vi "AN97005H-ONOFF.vi"(8 "error in":errorcluster caption="错误输入（无错误）", 10 "模式":enum16{"启动", "停止"}(ring), 11 "MyIndex":u8) -> (0 "error out":errorcluster caption="错误输出", 3 "OK?":bool)   [LabVIEW 2015, in "AN97005N.lvlib"]
uses:
  AN97005N.lvlib
  <vilib>/Instr/_visa.llb/VISA Configure Serial Port (Instr).vi
panel:
  out "AC电源":refnum<visa-resource-name>
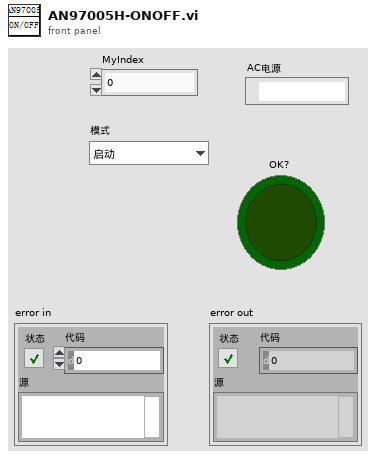
[diagram p1: front panel]
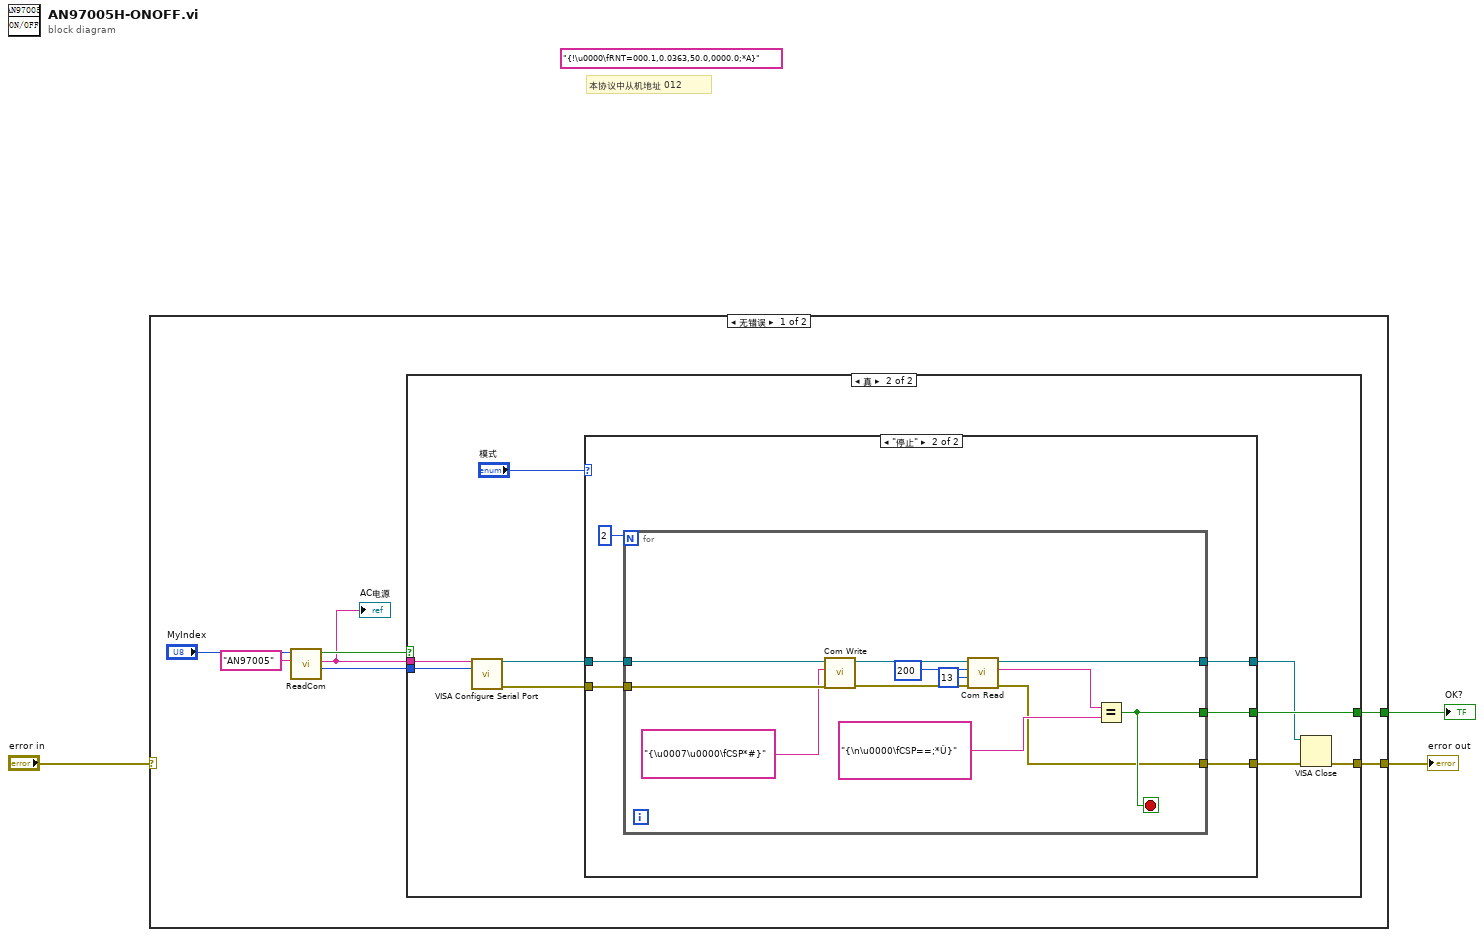
[diagram p0: block diagram]
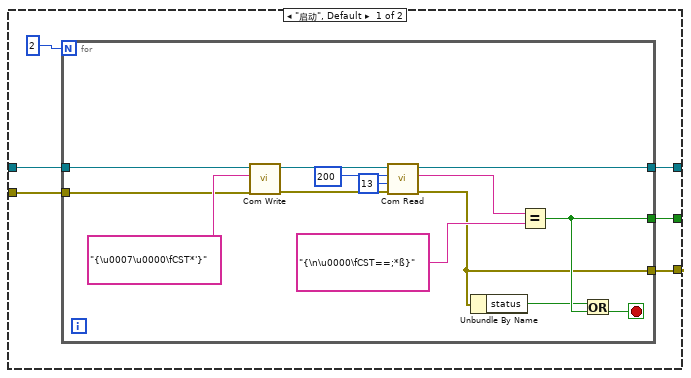
[diagram p3: hidden frame]
diagram:
  (unwired) "{!\u0000\fRNT=000.1,0.0363,50.0,0000.0;*A}"
  # "本协议中从机地址 012"
  n1 = case shown="无错误" "error in" {
    selector: "error in" -> [_ w58]
    tunnel: [w10 _] -> w3
    tunnel: [w4 w58] -> w2
    frame No Error {
      n2 = call "ReadCom.vi"("仪器名称"="AN97005", "MyIndex"="MyIndex") -> ("Baudrate"=w6:i32, "COM"=w5:string, "OK?"=w7:bool)  [unwired: 7 in]
      "AC电源" <- w5
      n3 = case shown="真" w7 {
        tunnel: [_ w18] -> w10
        tunnel: [_ w14] -> w4
        tunnel: w5 -> [_ w16]
        tunnel: w6 -> [_ w11]
        frame False {
        }
        frame True {
          n4 = call-poly "VISA Configure Serial Port"("VISA resource name"=w16, "baud rate (9600)"=w11) -> ("VISA resource name out"=w15:refnum<visa-resource-name>, "error out"=w12:errorcluster)  [unwired: 12 in]
          n5 = case shown="\"停止\"" "模式" {
            tunnel: w15 -> [w25 w45]
            tunnel: [w23 w43] -> w18
            tunnel: [w22 w42] -> w17
            tunnel: [w21 w41] -> w13
            tunnel: w12 -> [w20 w40]
            frame "启动", Default {
              n6 = for {
                N: 2 -> [_]
                tunnel: [w30] -> w23
                tunnel: [w29] -> w22
                tunnel: w25 -> [w39]
                tunnel: [w33] -> w21
                tunnel: w20 -> [w26]
                stop <- w28 stop-if-true
                n7 = call "Com Write.vi"("错误输入（无错误）"=w26, "Wbuff"="{\u0007\u0000\fCST*'}", "VISA In"=w39) -> ("错误输出"=w36:errorcluster, "VISA Out"=w37:refnum<visa-resource-name>)  [unwired: 7 in]
                n8 = call "Com Read.vi"("错误输入（无错误）"=w36, "num"=u32 13, "超时"=u32 200, "VISA In"=w37) -> ("错误输出"=w29:errorcluster, "buff"=w32:string, "VISA Out"=w33:refnum<visa-resource-name>)  [unwired: 5 in]
                n9 = Unbundle By Name(w29) -> ("status"=w27:bool)
                n10 = Equal?(x=w32, y="{\n\u0000\fCST==;*ß}" ("Wbuff")) -> (x = y?=w30:bool)
                n11 = Or(x=w27, y=w30) -> (x .or. y?=w28:bool)
              }
            }
            frame "停止" {
              n12 = for {
                N: 2 -> [_]
                tunnel: [w49] -> w43
                tunnel: [w48] -> w42
                tunnel: w45 -> [w57]
                tunnel: [w52] -> w41
                tunnel: w40 -> [w47]
                stop <- w49 stop-if-true
                n13 = call "Com Write.vi"("错误输入（无错误）"=w47, "Wbuff"="{\u0007\u0000\fCSP*#}", "VISA In"=w57) -> ("错误输出"=w55:errorcluster, "VISA Out"=w56:refnum<visa-resource-name>)  [unwired: 7 in]
                n14 = call "Com Read.vi"("错误输入（无错误）"=w55, "num"=u32 13, "超时"=u32 200, "VISA In"=w56) -> ("错误输出"=w48:errorcluster, "buff"=w51:string, "VISA Out"=w52:refnum<visa-resource-name>)  [unwired: 5 in]
                n15 = Equal?(x=w51, y="{\n\u0000\fCSP==;*Û}" ("Wbuff")) -> (x = y?=w49:bool)
              }
            }
          }
          n16 = VISA Close(VISA resource name=w13, error in (no error)=w17) -> (error out=w14:errorcluster)
        }
      }
    }
    frame Error {
    }
  }
  "OK?" <- w3
  "error out" <- w2
